vi "Auto_Throttle 01234.vi"(11 "Throttle":dbl(slide) scale=1.0..-1.0) -> (3 "01234":u16)   [LabVIEW 2016]
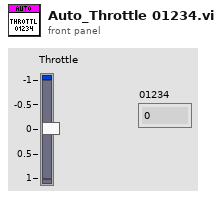
[diagram p1: front panel]
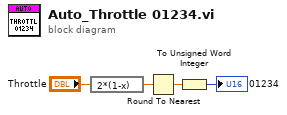
[diagram p0: block diagram]
diagram:
  n1 = expression code="2*(1-x)"("Throttle") -> (w4:dbl)
  n2 = Round To Nearest(number=w4) -> (nearest integer value=w2:dbl)
  n3 = To Unsigned Word Integer(number=w2) -> (unsigned 16bit integer=→"01234":u16)
